vi "DistPointLine.vi"(8 "P2":dbl[](array[numeric]), 9 "P1":dbl[](array[numeric]), 11 "Q":dbl[](array[numeric])) -> (2 "distance":dbl)   [LabVIEW 2023]
uses:
  <vilib>/Analysis/_algsub.llb/Real Vector Norm.vi
  <vilib>/Analysis/NI_AALPro.lvlib
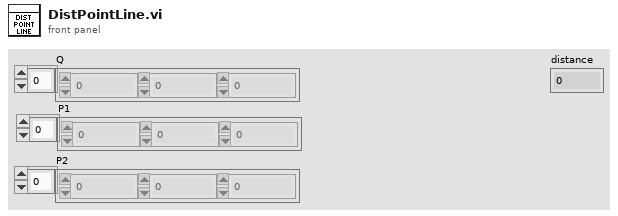
[diagram p1: front panel]
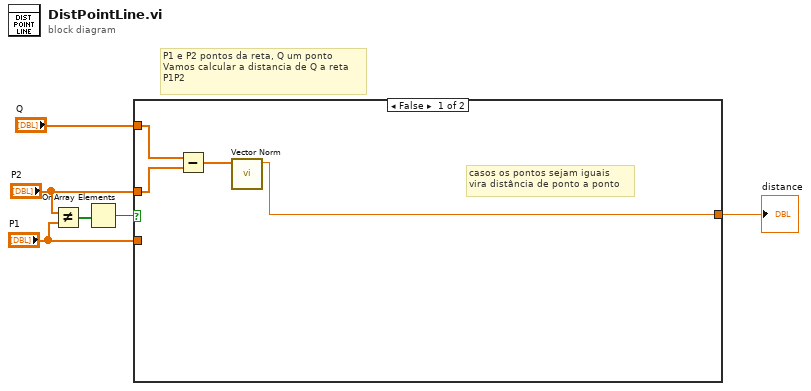
[diagram p0: block diagram]
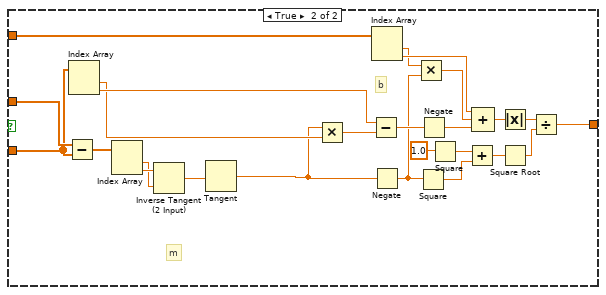
[diagram p2: hidden frame]
diagram:
  # "P1 e P2 pontos da reta, Q um ponto\nVamos calcular a distancia de Q a reta \nP1P2"
  n1 = Not Equal?(x="P2", y="P1") -> (x != y?=w2:bool[])
  n2 = Or Array Elements(Boolean array=w2) -> (logical OR=w1:bool)
  n3 = case shown="False" w1 {
    tunnel: "P2" -> [w9 w35]
    tunnel: "P1" -> [_ w31]
    tunnel: "Q" -> [w10 w27]
    tunnel: [w7 w13] -> w5
    frame False {
      # "casos os pontos sejam iguais\nvira distância de ponto a ponto"
      n4 = Subtract(x=w10, y=w9) -> (x-y=w8:dbl[])
      n5 = call-poly <vilib>:"Vector Norm.vi"("Input Vector"=w8) -> ("norm"=w7:dbl)  [unwired: 9 in, 1 out]
    }
    frame True {
      # "b"
      # "m"
      n6 = Subtract(x=w35, y=w31) -> (x-y=w34:dbl[])
      n7 = Index Array(array=w31) -> (element #1=w29:dbl, element #2=w30:dbl)  [unwired: 2 in]
      n8 = Index Array(array=w34) -> (element #1=w32:dbl, element #2=w33:dbl)  [unwired: 2 in]
      n9 = Inverse Tangent (2 Input)(1:w32, 2:w33) -> (0:w12:dbl)
      n10 = Tangent(1:w12) -> (0:w11:dbl)
      n11 = Multiply(x=w11, y=w29) -> (x*y=w28:dbl)
      n12 = Subtract(x=w30, y=w28) -> (x-y=w23:dbl)
      n13 = Index Array(array=w27) -> (element #1=w25:dbl, element #2=w26:dbl)  [unwired: 2 in]
      n14 = Negate(x=w11) -> (-x=w19:dbl)
      n15 = Multiply(x=w25, y=w19) -> (x*y=w24:dbl)
      n16 = Square(x=w19) -> (x^2=w17:dbl)
      n17 = Negate(x=w23) -> (-x=w22:dbl)
      n18 = Square(x=1.0) -> (x^2=w18:dbl)
      n19 = Add(x=w18, y=w17) -> (x+y=w16:dbl)
      n20 = Compound Arithmetic op=ADD(w26, w24, w22) -> (w21:dbl)
      n21 = Absolute Value(x=w21) -> (abs(x)=w15:dbl)
      n22 = Square Root(x=w16) -> (sqrt(x)=w14:dbl)
      n23 = Divide(x=w15, y=w14) -> (x/y=w13:dbl)
    }
  }
  "distance" <- w5
